vi "Main.vi"() -> ()   [LabVIEW 2021] (continued)
                n259 = Two Button Dialog(message="确定修改？" ("消息")) -> (T button?=w366:bool)  [unwired: 2 in]
                n260 = local read "控件配置文件"() -> (w364:string[][])
                n261 = property on="表格" class="Tbl (严格)"() -> ("Value"=w363:string[][])  [unwired: 2 in, 2 out]
                n262 = call "设控值写入.vi"("表格"=w363, "控件配置文件"=w364, "DataInitDef"=w361, "NewVal"=w365, "布尔"=w366) -> ("输出簇"=w362:cluster{u16, i32, i32, i32})  [unwired: 10 in]
                n263 = property on="要发送的数据" class="Clust (严格)"("Val(Sgnl)"=w362) -> ()  [unwired: 2 in, 2 out]
              }
              event "设控2": Value Change {
                w368 = T9 23 items=["刷新间隔", "波特率", "布尔1设置项", "布尔2设置项", "布尔3设置项", "布尔4设置项", "布尔5设置项", "布尔6设置项", "布尔7设置项", "布尔8设置项", "显控1设置", "显控2设置", "显控3设置", "显控4设置", "显控5设置", "显控6设置", "显控7设置", "显控8设置", "显控9设置", "显控10设置", "显控11设置", "显控12设置", "设控1设置", "设控2设置", "设控3设置", "设控4设置", "设控5设置", "设控6设置", "设控7设置", "设控8设置", "曲线1设置", "曲线2设置", "曲线3设置", "曲线4设置", "曲线5设置", "曲线6设置", "曲线7设置", "曲线8设置", "曲线9设置", "曲线10设置", "曲线11设置", "曲线12设置", "曲线13设置", "曲线14设置", "曲线15设置", "曲线16设置", "曲线17设置", "曲线18设置", "曲线19设置", "曲线20设置", "曲线21设置", "曲线22设置", "曲线23设置", "曲线24设置", "曲线25设置", "曲线26设置", "曲线27设置", "曲线28设置", "曲线29设置", "曲线30设置", "曲线31设置", "曲线32设置", "曲线33设置", "曲线34设置", "曲线35设置", "曲线36设置", "曲线37设置", "曲线38设置", "曲线39设置", "曲线40设置", "曲线41设置", "曲线42设置", "曲线43设置", "曲线44设置", "曲线45设置", "曲线46设置", "曲线47设置", "曲线48设置", "曲线49设置", "曲线50设置", "曲线51设置", "曲线52设置", "曲线53设置", "曲线54设置", "曲线55设置", "曲线56设置", "曲线57设置", "曲线58设置", "曲线59设置", "曲线60设置", "曲线61设置", "曲线62设置", "曲线63设置", "曲线64设置", "ID值", "数据模式"] ("DataInitDef")
                n264 = event-data() -> ("NewVal"=w370:string)  [unwired: 1 in, 5 out]
                n265 = Two Button Dialog(message="确定修改？" ("消息")) -> (T button?=w369:bool)  [unwired: 2 in]
                n266 = local read "控件配置文件"() -> (w371:string[][])
                n267 = property on="表格" class="Tbl (严格)"() -> ("Value"=w372:string[][])  [unwired: 2 in, 2 out]
                n268 = call "设控值写入.vi"("表格"=w372, "控件配置文件"=w371, "DataInitDef"=w368, "NewVal"=w370, "布尔"=w369) -> ("输出簇"=w373:cluster{u16, i32, i32, i32})  [unwired: 10 in]
                n269 = property on="要发送的数据" class="Clust (严格)"("Val(Sgnl)"=w373) -> ()  [unwired: 2 in, 2 out]
              }
              event "设控3": Value Change {
                w375 = T9 24 items=["刷新间隔", "波特率", "布尔1设置项", "布尔2设置项", "布尔3设置项", "布尔4设置项", "布尔5设置项", "布尔6设置项", "布尔7设置项", "布尔8设置项", "显控1设置", "显控2设置", "显控3设置", "显控4设置", "显控5设置", "显控6设置", "显控7设置", "显控8设置", "显控9设置", "显控10设置", "显控11设置", "显控12设置", "设控1设置", "设控2设置", "设控3设置", "设控4设置", "设控5设置", "设控6设置", "设控7设置", "设控8设置", "曲线1设置", "曲线2设置", "曲线3设置", "曲线4设置", "曲线5设置", "曲线6设置", "曲线7设置", "曲线8设置", "曲线9设置", "曲线10设置", "曲线11设置", "曲线12设置", "曲线13设置", "曲线14设置", "曲线15设置", "曲线16设置", "曲线17设置", "曲线18设置", "曲线19设置", "曲线20设置", "曲线21设置", "曲线22设置", "曲线23设置", "曲线24设置", "曲线25设置", "曲线26设置", "曲线27设置", "曲线28设置", "曲线29设置", "曲线30设置", "曲线31设置", "曲线32设置", "曲线33设置", "曲线34设置", "曲线35设置", "曲线36设置", "曲线37设置", "曲线38设置", "曲线39设置", "曲线40设置", "曲线41设置", "曲线42设置", "曲线43设置", "曲线44设置", "曲线45设置", "曲线46设置", "曲线47设置", "曲线48设置", "曲线49设置", "曲线50设置", "曲线51设置", "曲线52设置", "曲线53设置", "曲线54设置", "曲线55设置", "曲线56设置", "曲线57设置", "曲线58设置", "曲线59设置", "曲线60设置", "曲线61设置", "曲线62设置", "曲线63设置", "曲线64设置", "ID值", "数据模式"] ("DataInitDef")
                n270 = event-data() -> ("NewVal"=w378:string)  [unwired: 1 in, 5 out]
                n271 = Two Button Dialog(message="确定修改？" ("消息")) -> (T button?=w377:bool)  [unwired: 2 in]
                n272 = local read "控件配置文件"() -> (w379:string[][])
                n273 = property on="表格" class="Tbl (严格)"() -> ("Value"=w380:string[][])  [unwired: 2 in, 2 out]
                n274 = call "设控值写入.vi"("表格"=w380, "控件配置文件"=w379, "DataInitDef"=w375, "NewVal"=w378, "布尔"=w377) -> ("输出簇"=w376:cluster{u16, i32, i32, i32})  [unwired: 10 in]
                n275 = property on="要发送的数据" class="Clust (严格)"("Val(Sgnl)"=w376) -> ()  [unwired: 2 in, 2 out]
              }
              event "设控4": Value Change {
                w382 = T9 25 items=["刷新间隔", "波特率", "布尔1设置项", "布尔2设置项", "布尔3设置项", "布尔4设置项", "布尔5设置项", "布尔6设置项", "布尔7设置项", "布尔8设置项", "显控1设置", "显控2设置", "显控3设置", "显控4设置", "显控5设置", "显控6设置", "显控7设置", "显控8设置", "显控9设置", "显控10设置", "显控11设置", "显控12设置", "设控1设置", "设控2设置", "设控3设置", "设控4设置", "设控5设置", "设控6设置", "设控7设置", "设控8设置", "曲线1设置", "曲线2设置", "曲线3设置", "曲线4设置", "曲线5设置", "曲线6设置", "曲线7设置", "曲线8设置", "曲线9设置", "曲线10设置", "曲线11设置", "曲线12设置", "曲线13设置", "曲线14设置", "曲线15设置", "曲线16设置", "曲线17设置", "曲线18设置", "曲线19设置", "曲线20设置", "曲线21设置", "曲线22设置", "曲线23设置", "曲线24设置", "曲线25设置", "曲线26设置", "曲线27设置", "曲线28设置", "曲线29设置", "曲线30设置", "曲线31设置", "曲线32设置", "曲线33设置", "曲线34设置", "曲线35设置", "曲线36设置", "曲线37设置", "曲线38设置", "曲线39设置", "曲线40设置", "曲线41设置", "曲线42设置", "曲线43设置", "曲线44设置", "曲线45设置", "曲线46设置", "曲线47设置", "曲线48设置", "曲线49设置", "曲线50设置", "曲线51设置", "曲线52设置", "曲线53设置", "曲线54设置", "曲线55设置", "曲线56设置", "曲线57设置", "曲线58设置", "曲线59设置", "曲线60设置", "曲线61设置", "曲线62设置", "曲线63设置", "曲线64设置", "ID值", "数据模式"] ("DataInitDef")
                n276 = event-data() -> ("NewVal"=w385:string)  [unwired: 1 in, 5 out]
                n277 = Two Button Dialog(message="确定修改？" ("消息")) -> (T button?=w384:bool)  [unwired: 2 in]
                n278 = local read "控件配置文件"() -> (w386:string[][])
                n279 = property on="表格" class="Tbl (严格)"() -> ("Value"=w387:string[][])  [unwired: 2 in, 2 out]
                n280 = call "设控值写入.vi"("表格"=w387, "控件配置文件"=w386, "DataInitDef"=w382, "NewVal"=w385, "布尔"=w384) -> ("输出簇"=w383:cluster{u16, i32, i32, i32})  [unwired: 10 in]
                n281 = property on="要发送的数据" class="Clust (严格)"("Val(Sgnl)"=w383) -> ()  [unwired: 2 in, 2 out]
              }
              event "设控5": Value Change {
                w389 = T9 26 items=["刷新间隔", "波特率", "布尔1设置项", "布尔2设置项", "布尔3设置项", "布尔4设置项", "布尔5设置项", "布尔6设置项", "布尔7设置项", "布尔8设置项", "显控1设置", "显控2设置", "显控3设置", "显控4设置", "显控5设置", "显控6设置", "显控7设置", "显控8设置", "显控9设置", "显控10设置", "显控11设置", "显控12设置", "设控1设置", "设控2设置", "设控3设置", "设控4设置", "设控5设置", "设控6设置", "设控7设置", "设控8设置", "曲线1设置", "曲线2设置", "曲线3设置", "曲线4设置", "曲线5设置", "曲线6设置", "曲线7设置", "曲线8设置", "曲线9设置", "曲线10设置", "曲线11设置", "曲线12设置", "曲线13设置", "曲线14设置", "曲线15设置", "曲线16设置", "曲线17设置", "曲线18设置", "曲线19设置", "曲线20设置", "曲线21设置", "曲线22设置", "曲线23设置", "曲线24设置", "曲线25设置", "曲线26设置", "曲线27设置", "曲线28设置", "曲线29设置", "曲线30设置", "曲线31设置", "曲线32设置", "曲线33设置", "曲线34设置", "曲线35设置", "曲线36设置", "曲线37设置", "曲线38设置", "曲线39设置", "曲线40设置", "曲线41设置", "曲线42设置", "曲线43设置", "曲线44设置", "曲线45设置", "曲线46设置", "曲线47设置", "曲线48设置", "曲线49设置", "曲线50设置", "曲线51设置", "曲线52设置", "曲线53设置", "曲线54设置", "曲线55设置", "曲线56设置", "曲线57设置", "曲线58设置", "曲线59设置", "曲线60设置", "曲线61设置", "曲线62设置", "曲线63设置", "曲线64设置", "ID值", "数据模式"] ("DataInitDef")
                n282 = event-data() -> ("NewVal"=w391:string)  [unwired: 1 in, 5 out]
                n283 = Two Button Dialog(message="确定修改？" ("消息")) -> (T button?=w390:bool)  [unwired: 2 in]
                n284 = local read "控件配置文件"() -> (w392:string[][])
                n285 = property on="表格" class="Tbl (严格)"() -> ("Value"=w393:string[][])  [unwired: 2 in, 2 out]
                n286 = call "设控值写入.vi"("表格"=w393, "控件配置文件"=w392, "DataInitDef"=w389, "NewVal"=w391, "布尔"=w390) -> ("输出簇"=w394:cluster{u16, i32, i32, i32})  [unwired: 10 in]
                n287 = property on="要发送的数据" class="Clust (严格)"("Val(Sgnl)"=w394) -> ()  [unwired: 2 in, 2 out]
              }
              event "设控6": Value Change {
                w396 = T9 27 items=["刷新间隔", "波特率", "布尔1设置项", "布尔2设置项", "布尔3设置项", "布尔4设置项", "布尔5设置项", "布尔6设置项", "布尔7设置项", "布尔8设置项", "显控1设置", "显控2设置", "显控3设置", "显控4设置", "显控5设置", "显控6设置", "显控7设置", "显控8设置", "显控9设置", "显控10设置", "显控11设置", "显控12设置", "设控1设置", "设控2设置", "设控3设置", "设控4设置", "设控5设置", "设控6设置", "设控7设置", "设控8设置", "曲线1设置", "曲线2设置", "曲线3设置", "曲线4设置", "曲线5设置", "曲线6设置", "曲线7设置", "曲线8设置", "曲线9设置", "曲线10设置", "曲线11设置", "曲线12设置", "曲线13设置", "曲线14设置", "曲线15设置", "曲线16设置", "曲线17设置", "曲线18设置", "曲线19设置", "曲线20设置", "曲线21设置", "曲线22设置", "曲线23设置", "曲线24设置", "曲线25设置", "曲线26设置", "曲线27设置", "曲线28设置", "曲线29设置", "曲线30设置", "曲线31设置", "曲线32设置", "曲线33设置", "曲线34设置", "曲线35设置", "曲线36设置", "曲线37设置", "曲线38设置", "曲线39设置", "曲线40设置", "曲线41设置", "曲线42设置", "曲线43设置", "曲线44设置", "曲线45设置", "曲线46设置", "曲线47设置", "曲线48设置", "曲线49设置", "曲线50设置", "曲线51设置", "曲线52设置", "曲线53设置", "曲线54设置", "曲线55设置", "曲线56设置", "曲线57设置", "曲线58设置", "曲线59设置", "曲线60设置", "曲线61设置", "曲线62设置", "曲线63设置", "曲线64设置", "ID值", "数据模式"] ("DataInitDef")
                n288 = event-data() -> ("NewVal"=w398:string)  [unwired: 1 in, 5 out]
                n289 = Two Button Dialog(message="确定修改？" ("消息")) -> (T button?=w397:bool)  [unwired: 2 in]
                n290 = local read "控件配置文件"() -> (w399:string[][])
                n291 = property on="表格" class="Tbl (严格)"() -> ("Value"=w400:string[][])  [unwired: 2 in, 2 out]
                n292 = call "设控值写入.vi"("表格"=w400, "控件配置文件"=w399, "DataInitDef"=w396, "NewVal"=w398, "布尔"=w397) -> ("输出簇"=w401:cluster{u16, i32, i32, i32})  [unwired: 10 in]
                n293 = property on="要发送的数据" class="Clust (严格)"("Val(Sgnl)"=w401) -> ()  [unwired: 2 in, 2 out]
              }
              event "设控7": Value Change {
                w403 = T9 28 items=["刷新间隔", "波特率", "布尔1设置项", "布尔2设置项", "布尔3设置项", "布尔4设置项", "布尔5设置项", "布尔6设置项", "布尔7设置项", "布尔8设置项", "显控1设置", "显控2设置", "显控3设置", "显控4设置", "显控5设置", "显控6设置", "显控7设置", "显控8设置", "显控9设置", "显控10设置", "显控11设置", "显控12设置", "设控1设置", "设控2设置", "设控3设置", "设控4设置", "设控5设置", "设控6设置", "设控7设置", "设控8设置", "曲线1设置", "曲线2设置", "曲线3设置", "曲线4设置", "曲线5设置", "曲线6设置", "曲线7设置", "曲线8设置", "曲线9设置", "曲线10设置", "曲线11设置", "曲线12设置", "曲线13设置", "曲线14设置", "曲线15设置", "曲线16设置", "曲线17设置", "曲线18设置", "曲线19设置", "曲线20设置", "曲线21设置", "曲线22设置", "曲线23设置", "曲线24设置", "曲线25设置", "曲线26设置", "曲线27设置", "曲线28设置", "曲线29设置", "曲线30设置", "曲线31设置", "曲线32设置", "曲线33设置", "曲线34设置", "曲线35设置", "曲线36设置", "曲线37设置", "曲线38设置", "曲线39设置", "曲线40设置", "曲线41设置", "曲线42设置", "曲线43设置", "曲线44设置", "曲线45设置", "曲线46设置", "曲线47设置", "曲线48设置", "曲线49设置", "曲线50设置", "曲线51设置", "曲线52设置", "曲线53设置", "曲线54设置", "曲线55设置", "曲线56设置", "曲线57设置", "曲线58设置", "曲线59设置", "曲线60设置", "曲线61设置", "曲线62设置", "曲线63设置", "曲线64设置", "ID值", "数据模式"] ("DataInitDef")
                n294 = event-data() -> ("NewVal"=w405:string)  [unwired: 1 in, 5 out]
                n295 = Two Button Dialog(message="确定修改？" ("消息")) -> (T button?=w404:bool)  [unwired: 2 in]
                n296 = local read "控件配置文件"() -> (w406:string[][])
                n297 = property on="表格" class="Tbl (严格)"() -> ("Value"=w407:string[][])  [unwired: 2 in, 2 out]
                n298 = call "设控值写入.vi"("表格"=w407, "控件配置文件"=w406, "DataInitDef"=w403, "NewVal"=w405, "布尔"=w404) -> ("输出簇"=w408:cluster{u16, i32, i32, i32})  [unwired: 10 in]
                n299 = property on="要发送的数据" class="Clust (严格)"("Val(Sgnl)"=w408) -> ()  [unwired: 2 in, 2 out]
              }
              event "设控8": Value Change {
                w410 = T9 29 items=["刷新间隔", "波特率", "布尔1设置项", "布尔2设置项", "布尔3设置项", "布尔4设置项", "布尔5设置项", "布尔6设置项", "布尔7设置项", "布尔8设置项", "显控1设置", "显控2设置", "显控3设置", "显控4设置", "显控5设置", "显控6设置", "显控7设置", "显控8设置", "显控9设置", "显控10设置", "显控11设置", "显控12设置", "设控1设置", "设控2设置", "设控3设置", "设控4设置", "设控5设置", "设控6设置", "设控7设置", "设控8设置", "曲线1设置", "曲线2设置", "曲线3设置", "曲线4设置", "曲线5设置", "曲线6设置", "曲线7设置", "曲线8设置", "曲线9设置", "曲线10设置", "曲线11设置", "曲线12设置", "曲线13设置", "曲线14设置", "曲线15设置", "曲线16设置", "曲线17设置", "曲线18设置", "曲线19设置", "曲线20设置", "曲线21设置", "曲线22设置", "曲线23设置", "曲线24设置", "曲线25设置", "曲线26设置", "曲线27设置", "曲线28设置", "曲线29设置", "曲线30设置", "曲线31设置", "曲线32设置", "曲线33设置", "曲线34设置", "曲线35设置", "曲线36设置", "曲线37设置", "曲线38设置", "曲线39设置", "曲线40设置", "曲线41设置", "曲线42设置", "曲线43设置", "曲线44设置", "曲线45设置", "曲线46设置", "曲线47设置", "曲线48设置", "曲线49设置", "曲线50设置", "曲线51设置", "曲线52设置", "曲线53设置", "曲线54设置", "曲线55设置", "曲线56设置", "曲线57设置", "曲线58设置", "曲线59设置", "曲线60设置", "曲线61设置", "曲线62设置", "曲线63设置", "曲线64设置", "ID值", "数据模式"] ("DataInitDef")
                n300 = event-data() -> ("NewVal"=w412:string)  [unwired: 1 in, 5 out]
                n301 = Two Button Dialog(message="确定修改？" ("消息")) -> (T button?=w411:bool)  [unwired: 2 in]
                n302 = local read "控件配置文件"() -> (w413:string[][])
                n303 = property on="表格" class="Tbl (严格)"() -> ("Value"=w414:string[][])  [unwired: 2 in, 2 out]
                n304 = call "设控值写入.vi"("表格"=w414, "控件配置文件"=w413, "DataInitDef"=w410, "NewVal"=w412, "布尔"=w411) -> ("输出簇"=w415:cluster{u16, i32, i32, i32})  [unwired: 10 in]
                n305 = property on="要发送的数据" class="Clust (严格)"("Val(Sgnl)"=w415) -> ()  [unwired: 2 in, 2 out]
              }
              event "布尔 2": Value Change {
                w417 = T9 3 items=["刷新间隔", "波特率", "布尔1设置项", "布尔2设置项", "布尔3设置项", "布尔4设置项", "布尔5设置项", "布尔6设置项", "布尔7设置项", "布尔8设置项", "显控1设置", "显控2设置", "显控3设置", "显控4设置", "显控5设置", "显控6设置", "显控7设置", "显控8设置", "显控9设置", "显控10设置", "显控11设置", "显控12设置", "设控1设置", "设控2设置", "设控3设置", "设控4设置", "设控5设置", "设控6设置", "设控7设置", "设控8设置", "曲线1设置", "曲线2设置", "曲线3设置", "曲线4设置", "曲线5设置", "曲线6设置", "曲线7设置", "曲线8设置", "曲线9设置", "曲线10设置", "曲线11设置", "曲线12设置", "曲线13设置", "曲线14设置", "曲线15设置", "曲线16设置", "曲线17设置", "曲线18设置", "曲线19设置", "曲线20设置", "曲线21设置", "曲线22设置", "曲线23设置", "曲线24设置", "曲线25设置", "曲线26设置", "曲线27设置", "曲线28设置", "曲线29设置", "曲线30设置", "曲线31设置", "曲线32设置", "曲线33设置", "曲线34设置", "曲线35设置", "曲线36设置", "曲线37设置", "曲线38设置", "曲线39设置", "曲线40设置", "曲线41设置", "曲线42设置", "曲线43设置", "曲线44设置", "曲线45设置", "曲线46设置", "曲线47设置", "曲线48设置", "曲线49设置", "曲线50设置", "曲线51设置", "曲线52设置", "曲线53设置", "曲线54设置", "曲线55设置", "曲线56设置", "曲线57设置", "曲线58设置", "曲线59设置", "曲线60设置", "曲线61设置", "曲线62设置", "曲线63设置", "曲线64设置", "ID值", "数据模式"] ("DataInitDef")
                n306 = event-data() -> ("NewVal"=w418:bool)  [unwired: 1 in]
                n307 = local read "控件配置文件"() -> (w424:string[][])
                n308 = Index Array(array=w424, index (row)=w417, index (col)=1 ("禁用的索引 (列)")) -> (element=w423:string)
                n309 = Not Equal?(x=w423, y="") -> (x != y?=w420:bool)
                n310 = Not Equal?(x=w423, y="X") -> (x != y?=w419:bool)
                n311 = And(x=w420, y=w419) -> (x .and. y?=w421:bool)
                n312 = case shown="真" w421 {
                  tunnel: w418 -> [_ w428]
                  tunnel: w423 -> [_ w429]
                  frame False {
                  }
                  frame True {
                    n313 = local write "延时更新布尔状态"(i16 0 ("延时更新布尔状态")) -> ()
                    n314 = property on="表格" class="Tbl (严格)"() -> ("Value"=w430:string[][])  [unwired: 2 in, 2 out]
                    n315 = call "布尔数据处理.vi"("布尔输入"=w428, "行数"=w429, "表格"=w430) -> ("要发送的数据"=w427:cluster{"地址":u16, "数据":i32, "行数":i32, "ID":i32})  [unwired: 8 in]
                    n316 = property on="要发送的数据" class="Clust (严格)"("Val(Sgnl)"=w427) -> ()  [unwired: 2 in, 2 out]
                  }
                }
              }
              event "布尔 3": Value Change {
                w432 = T9 4 items=["刷新间隔", "波特率", "布尔1设置项", "布尔2设置项", "布尔3设置项", "布尔4设置项", "布尔5设置项", "布尔6设置项", "布尔7设置项", "布尔8设置项", "显控1设置", "显控2设置", "显控3设置", "显控4设置", "显控5设置", "显控6设置", "显控7设置", "显控8设置", "显控9设置", "显控10设置", "显控11设置", "显控12设置", "设控1设置", "设控2设置", "设控3设置", "设控4设置", "设控5设置", "设控6设置", "设控7设置", "设控8设置", "曲线1设置", "曲线2设置", "曲线3设置", "曲线4设置", "曲线5设置", "曲线6设置", "曲线7设置", "曲线8设置", "曲线9设置", "曲线10设置", "曲线11设置", "曲线12设置", "曲线13设置", "曲线14设置", "曲线15设置", "曲线16设置", "曲线17设置", "曲线18设置", "曲线19设置", "曲线20设置", "曲线21设置", "曲线22设置", "曲线23设置", "曲线24设置", "曲线25设置", "曲线26设置", "曲线27设置", "曲线28设置", "曲线29设置", "曲线30设置", "曲线31设置", "曲线32设置", "曲线33设置", "曲线34设置", "曲线35设置", "曲线36设置", "曲线37设置", "曲线38设置", "曲线39设置", "曲线40设置", "曲线41设置", "曲线42设置", "曲线43设置", "曲线44设置", "曲线45设置", "曲线46设置", "曲线47设置", "曲线48设置", "曲线49设置", "曲线50设置", "曲线51设置", "曲线52设置", "曲线53设置", "曲线54设置", "曲线55设置", "曲线56设置", "曲线57设置", "曲线58设置", "曲线59设置", "曲线60设置", "曲线61设置", "曲线62设置", "曲线63设置", "曲线64设置", "ID值", "数据模式"] ("DataInitDef")
                n317 = event-data() -> ("NewVal"=w433:bool)  [unwired: 1 in]
                n318 = local read "控件配置文件"() -> (w439:string[][])
                n319 = Index Array(array=w439, index (row)=w432, index (col)=1 ("禁用的索引 (列)")) -> (element=w438:string)
                n320 = Not Equal?(x=w438, y="") -> (x != y?=w435:bool)
                n321 = Not Equal?(x=w438, y="X") -> (x != y?=w434:bool)
                n322 = And(x=w435, y=w434) -> (x .and. y?=w436:bool)
                n323 = case shown="真" w436 {
                  tunnel: w438 -> [_ w444]
                  tunnel: w433 -> [_ w443]
                  frame False {
                  }
                  frame True {
                    n324 = local write "延时更新布尔状态"(i16 0 ("延时更新布尔状态")) -> ()
                    n325 = property on="表格" class="Tbl (严格)"() -> ("Value"=w445:string[][])  [unwired: 2 in, 2 out]
                    n326 = call "布尔数据处理.vi"("布尔输入"=w443, "行数"=w444, "表格"=w445) -> ("要发送的数据"=w442:cluster{"地址":u16, "数据":i32, "行数":i32, "ID":i32})  [unwired: 8 in]
                    n327 = property on="要发送的数据" class="Clust (严格)"("Val(Sgnl)"=w442) -> ()  [unwired: 2 in, 2 out]
                  }
                }
              }
              event "布尔 4": Value Change {
                w447 = T9 5 items=["刷新间隔", "波特率", "布尔1设置项", "布尔2设置项", "布尔3设置项", "布尔4设置项", "布尔5设置项", "布尔6设置项", "布尔7设置项", "布尔8设置项", "显控1设置", "显控2设置", "显控3设置", "显控4设置", "显控5设置", "显控6设置", "显控7设置", "显控8设置", "显控9设置", "显控10设置", "显控11设置", "显控12设置", "设控1设置", "设控2设置", "设控3设置", "设控4设置", "设控5设置", "设控6设置", "设控7设置", "设控8设置", "曲线1设置", "曲线2设置", "曲线3设置", "曲线4设置", "曲线5设置", "曲线6设置", "曲线7设置", "曲线8设置", "曲线9设置", "曲线10设置", "曲线11设置", "曲线12设置", "曲线13设置", "曲线14设置", "曲线15设置", "曲线16设置", "曲线17设置", "曲线18设置", "曲线19设置", "曲线20设置", "曲线21设置", "曲线22设置", "曲线23设置", "曲线24设置", "曲线25设置", "曲线26设置", "曲线27设置", "曲线28设置", "曲线29设置", "曲线30设置", "曲线31设置", "曲线32设置", "曲线33设置", "曲线34设置", "曲线35设置", "曲线36设置", "曲线37设置", "曲线38设置", "曲线39设置", "曲线40设置", "曲线41设置", "曲线42设置", "曲线43设置", "曲线44设置", "曲线45设置", "曲线46设置", "曲线47设置", "曲线48设置", "曲线49设置", "曲线50设置", "曲线51设置", "曲线52设置", "曲线53设置", "曲线54设置", "曲线55设置", "曲线56设置", "曲线57设置", "曲线58设置", "曲线59设置", "曲线60设置", "曲线61设置", "曲线62设置", "曲线63设置", "曲线64设置", "ID值", "数据模式"] ("DataInitDef")
                n328 = event-data() -> ("NewVal"=w448:bool)  [unwired: 1 in]
                n329 = local read "控件配置文件"() -> (w456:string[][])
                n330 = Index Array(array=w456, index (row)=w447, index (col)=1 ("禁用的索引 (列)")) -> (element=w455:string)
                n331 = Not Equal?(x=w455, y="") -> (x != y?=w453:bool)
                n332 = Not Equal?(x=w455, y="X") -> (x != y?=w452:bool)
                n333 = And(x=w453, y=w452) -> (x .and. y?=w454:bool)
                n334 = case shown="真" w454 {
                  tunnel: w448 -> [_ w458]
                  tunnel: w455 -> [_ w459]
                  frame False {
                  }
                  frame True {
                    n335 = local write "延时更新布尔状态"(i16 0 ("延时更新布尔状态")) -> ()
                    n336 = property on="表格" class="Tbl (严格)"() -> ("Value"=w460:string[][])  [unwired: 2 in, 2 out]
                    n337 = call "布尔数据处理.vi"("布尔输入"=w458, "行数"=w459, "表格"=w460) -> ("要发送的数据"=w457:cluster{"地址":u16, "数据":i32, "行数":i32, "ID":i32})  [unwired: 8 in]
                    n338 = property on="要发送的数据" class="Clust (严格)"("Val(Sgnl)"=w457) -> ()  [unwired: 2 in, 2 out]
                  }
                }
              }
              event "布尔 5": Value Change {
                w462 = T9 6 items=["刷新间隔", "波特率", "布尔1设置项", "布尔2设置项", "布尔3设置项", "布尔4设置项", "布尔5设置项", "布尔6设置项", "布尔7设置项", "布尔8设置项", "显控1设置", "显控2设置", "显控3设置", "显控4设置", "显控5设置", "显控6设置", "显控7设置", "显控8设置", "显控9设置", "显控10设置", "显控11设置", "显控12设置", "设控1设置", "设控2设置", "设控3设置", "设控4设置", "设控5设置", "设控6设置", "设控7设置", "设控8设置", "曲线1设置", "曲线2设置", "曲线3设置", "曲线4设置", "曲线5设置", "曲线6设置", "曲线7设置", "曲线8设置", "曲线9设置", "曲线10设置", "曲线11设置", "曲线12设置", "曲线13设置", "曲线14设置", "曲线15设置", "曲线16设置", "曲线17设置", "曲线18设置", "曲线19设置", "曲线20设置", "曲线21设置", "曲线22设置", "曲线23设置", "曲线24设置", "曲线25设置", "曲线26设置", "曲线27设置", "曲线28设置", "曲线29设置", "曲线30设置", "曲线31设置", "曲线32设置", "曲线33设置", "曲线34设置", "曲线35设置", "曲线36设置", "曲线37设置", "曲线38设置", "曲线39设置", "曲线40设置", "曲线41设置", "曲线42设置", "曲线43设置", "曲线44设置", "曲线45设置", "曲线46设置", "曲线47设置", "曲线48设置", "曲线49设置", "曲线50设置", "曲线51设置", "曲线52设置", "曲线53设置", "曲线54设置", "曲线55设置", "曲线56设置", "曲线57设置", "曲线58设置", "曲线59设置", "曲线60设置", "曲线61设置", "曲线62设置", "曲线63设置", "曲线64设置", "ID值", "数据模式"] ("DataInitDef")
                n339 = event-data() -> ("NewVal"=w463:bool)  [unwired: 1 in]
                n340 = local read "控件配置文件"() -> (w471:string[][])
                n341 = Index Array(array=w471, index (row)=w462, index (col)=1 ("禁用的索引 (列)")) -> (element=w470:string)
                n342 = Not Equal?(x=w470, y="") -> (x != y?=w468:bool)
                n343 = Not Equal?(x=w470, y="X") -> (x != y?=w467:bool)
                n344 = And(x=w468, y=w467) -> (x .and. y?=w469:bool)
                n345 = case shown="真" w469 {
                  tunnel: w463 -> [_ w473]
                  tunnel: w470 -> [_ w474]
                  frame False {
                  }
                  frame True {
                    n346 = local write "延时更新布尔状态"(i16 0 ("延时更新布尔状态")) -> ()
                    n347 = property on="表格" class="Tbl (严格)"() -> ("Value"=w475:string[][])  [unwired: 2 in, 2 out]
                    n348 = call "布尔数据处理.vi"("布尔输入"=w473, "行数"=w474, "表格"=w475) -> ("要发送的数据"=w472:cluster{"地址":u16, "数据":i32, "行数":i32, "ID":i32})  [unwired: 8 in]
                    n349 = property on="要发送的数据" class="Clust (严格)"("Val(Sgnl)"=w472) -> ()  [unwired: 2 in, 2 out]
                  }
                }
              }
              event "布尔 6": Value Change {
                w477 = T9 7 items=["刷新间隔", "波特率", "布尔1设置项", "布尔2设置项", "布尔3设置项", "布尔4设置项", "布尔5设置项", "布尔6设置项", "布尔7设置项", "布尔8设置项", "显控1设置", "显控2设置", "显控3设置", "显控4设置", "显控5设置", "显控6设置", "显控7设置", "显控8设置", "显控9设置", "显控10设置", "显控11设置", "显控12设置", "设控1设置", "设控2设置", "设控3设置", "设控4设置", "设控5设置", "设控6设置", "设控7设置", "设控8设置", "曲线1设置", "曲线2设置", "曲线3设置", "曲线4设置", "曲线5设置", "曲线6设置", "曲线7设置", "曲线8设置", "曲线9设置", "曲线10设置", "曲线11设置", "曲线12设置", "曲线13设置", "曲线14设置", "曲线15设置", "曲线16设置", "曲线17设置", "曲线18设置", "曲线19设置", "曲线20设置", "曲线21设置", "曲线22设置", "曲线23设置", "曲线24设置", "曲线25设置", "曲线26设置", "曲线27设置", "曲线28设置", "曲线29设置", "曲线30设置", "曲线31设置", "曲线32设置", "曲线33设置", "曲线34设置", "曲线35设置", "曲线36设置", "曲线37设置", "曲线38设置", "曲线39设置", "曲线40设置", "曲线41设置", "曲线42设置", "曲线43设置", "曲线44设置", "曲线45设置", "曲线46设置", "曲线47设置", "曲线48设置", "曲线49设置", "曲线50设置", "曲线51设置", "曲线52设置", "曲线53设置", "曲线54设置", "曲线55设置", "曲线56设置", "曲线57设置", "曲线58设置", "曲线59设置", "曲线60设置", "曲线61设置", "曲线62设置", "曲线63设置", "曲线64设置", "ID值", "数据模式"] ("DataInitDef")
                n350 = event-data() -> ("NewVal"=w478:bool)  [unwired: 1 in]
                n351 = local read "控件配置文件"() -> (w486:string[][])
                n352 = Index Array(array=w486, index (row)=w477, index (col)=1 ("禁用的索引 (列)")) -> (element=w485:string)
                n353 = Not Equal?(x=w485, y="") -> (x != y?=w483:bool)
                n354 = Not Equal?(x=w485, y="X") -> (x != y?=w482:bool)
                n355 = And(x=w483, y=w482) -> (x .and. y?=w484:bool)
                n356 = case shown="真" w484 {
                  tunnel: w478 -> [_ w488]
                  tunnel: w485 -> [_ w489]
                  frame False {
                  }
                  frame True {
                    n357 = local write "延时更新布尔状态"(i16 0 ("延时更新布尔状态")) -> ()
                    n358 = property on="表格" class="Tbl (严格)"() -> ("Value"=w490:string[][])  [unwired: 2 in, 2 out]
                    n359 = call "布尔数据处理.vi"("布尔输入"=w488, "行数"=w489, "表格"=w490) -> ("要发送的数据"=w487:cluster{"地址":u16, "数据":i32, "行数":i32, "ID":i32})  [unwired: 8 in]
                    n360 = property on="要发送的数据" class="Clust (严格)"("Val(Sgnl)"=w487) -> ()  [unwired: 2 in, 2 out]
                  }
                }
              }
              event "布尔 7": Value Change {
                w492 = T9 8 items=["刷新间隔", "波特率", "布尔1设置项", "布尔2设置项", "布尔3设置项", "布尔4设置项", "布尔5设置项", "布尔6设置项", "布尔7设置项", "布尔8设置项", "显控1设置", "显控2设置", "显控3设置", "显控4设置", "显控5设置", "显控6设置", "显控7设置", "显控8设置", "显控9设置", "显控10设置", "显控11设置", "显控12设置", "设控1设置", "设控2设置", "设控3设置", "设控4设置", "设控5设置", "设控6设置", "设控7设置", "设控8设置", "曲线1设置", "曲线2设置", "曲线3设置", "曲线4设置", "曲线5设置", "曲线6设置", "曲线7设置", "曲线8设置", "曲线9设置", "曲线10设置", "曲线11设置", "曲线12设置", "曲线13设置", "曲线14设置", "曲线15设置", "曲线16设置", "曲线17设置", "曲线18设置", "曲线19设置", "曲线20设置", "曲线21设置", "曲线22设置", "曲线23设置", "曲线24设置", "曲线25设置", "曲线26设置", "曲线27设置", "曲线28设置", "曲线29设置", "曲线30设置", "曲线31设置", "曲线32设置", "曲线33设置", "曲线34设置", "曲线35设置", "曲线36设置", "曲线37设置", "曲线38设置", "曲线39设置", "曲线40设置", "曲线41设置", "曲线42设置", "曲线43设置", "曲线44设置", "曲线45设置", "曲线46设置", "曲线47设置", "曲线48设置", "曲线49设置", "曲线50设置", "曲线51设置", "曲线52设置", "曲线53设置", "曲线54设置", "曲线55设置", "曲线56设置", "曲线57设置", "曲线58设置", "曲线59设置", "曲线60设置", "曲线61设置", "曲线62设置", "曲线63设置", "曲线64设置", "ID值", "数据模式"] ("DataInitDef")
                n361 = event-data() -> ("NewVal"=w493:bool)  [unwired: 1 in]
                n362 = local read "控件配置文件"() -> (w501:string[][])
                n363 = Index Array(array=w501, index (row)=w492, index (col)=1 ("禁用的索引 (列)")) -> (element=w500:string)
                n364 = Not Equal?(x=w500, y="") -> (x != y?=w498:bool)
                n365 = Not Equal?(x=w500, y="X") -> (x != y?=w497:bool)
                n366 = And(x=w498, y=w497) -> (x .and. y?=w499:bool)
                n367 = case shown="真" w499 {
                  tunnel: w493 -> [_ w503]
                  tunnel: w500 -> [_ w504]
                  frame False {
                  }
                  frame True {
                    n368 = local write "延时更新布尔状态"(i16 0 ("延时更新布尔状态")) -> ()
                    n369 = property on="表格" class="Tbl (严格)"() -> ("Value"=w505:string[][])  [unwired: 2 in, 2 out]
                    n370 = call "布尔数据处理.vi"("布尔输入"=w503, "行数"=w504, "表格"=w505) -> ("要发送的数据"=w502:cluster{"地址":u16, "数据":i32, "行数":i32, "ID":i32})  [unwired: 8 in]
                    n371 = property on="要发送的数据" class="Clust (严格)"("Val(Sgnl)"=w502) -> ()  [unwired: 2 in, 2 out]
                  }
                }
              }
              event "布尔 8": Value Change {
                w507 = T9 9 items=["刷新间隔", "波特率", "布尔1设置项", "布尔2设置项", "布尔3设置项", "布尔4设置项", "布尔5设置项", "布尔6设置项", "布尔7设置项", "布尔8设置项", "显控1设置", "显控2设置", "显控3设置", "显控4设置", "显控5设置", "显控6设置", "显控7设置", "显控8设置", "显控9设置", "显控10设置", "显控11设置", "显控12设置", "设控1设置", "设控2设置", "设控3设置", "设控4设置", "设控5设置", "设控6设置", "设控7设置", "设控8设置", "曲线1设置", "曲线2设置", "曲线3设置", "曲线4设置", "曲线5设置", "曲线6设置", "曲线7设置", "曲线8设置", "曲线9设置", "曲线10设置", "曲线11设置", "曲线12设置", "曲线13设置", "曲线14设置", "曲线15设置", "曲线16设置", "曲线17设置", "曲线18设置", "曲线19设置", "曲线20设置", "曲线21设置", "曲线22设置", "曲线23设置", "曲线24设置", "曲线25设置", "曲线26设置", "曲线27设置", "曲线28设置", "曲线29设置", "曲线30设置", "曲线31设置", "曲线32设置", "曲线33设置", "曲线34设置", "曲线35设置", "曲线36设置", "曲线37设置", "曲线38设置", "曲线39设置", "曲线40设置", "曲线41设置", "曲线42设置", "曲线43设置", "曲线44设置", "曲线45设置", "曲线46设置", "曲线47设置", "曲线48设置", "曲线49设置", "曲线50设置", "曲线51设置", "曲线52设置", "曲线53设置", "曲线54设置", "曲线55设置", "曲线56设置", "曲线57设置", "曲线58设置", "曲线59设置", "曲线60设置", "曲线61设置", "曲线62设置", "曲线63设置", "曲线64设置", "ID值", "数据模式"] ("DataInitDef")
                n372 = event-data() -> ("NewVal"=w508:bool)  [unwired: 1 in]
                n373 = local read "控件配置文件"() -> (w516:string[][])
                n374 = Index Array(array=w516, index (row)=w507, index (col)=1 ("禁用的索引 (列)")) -> (element=w515:string)
                n375 = Not Equal?(x=w515, y="") -> (x != y?=w513:bool)
                n376 = Not Equal?(x=w515, y="X") -> (x != y?=w512:bool)
                n377 = And(x=w513, y=w512) -> (x .and. y?=w514:bool)
                n378 = case shown="真" w514 {
                  tunnel: w508 -> [_ w518]
                  tunnel: w515 -> [_ w519]
                  frame False {
                  }
                  frame True {
                    n379 = local write "延时更新布尔状态"(i16 0 ("延时更新布尔状态")) -> ()
                    n380 = property on="表格" class="Tbl (严格)"() -> ("Value"=w520:string[][])  [unwired: 2 in, 2 out]
                    n381 = call "布尔数据处理.vi"("布尔输入"=w518, "行数"=w519, "表格"=w520) -> ("要发送的数据"=w517:cluster{"地址":u16, "数据":i32, "行数":i32, "ID":i32})  [unwired: 8 in]
                    n382 = property on="要发送的数据" class="Clust (严格)"("Val(Sgnl)"=w517) -> ()  [unwired: 2 in, 2 out]
                  }
                }
              }
            }
          }
          frame #1 {
            # "处理表格右键关联的代码"
            n383 = event "事件结构" shown="[1] \"表格\": 快捷菜单选择（用户）" {
              selector: _ -> [_ _]
              dyn-events: _ -> [_ _]
              timeout: 0 -> [_ _]
              event Timeout {
                n384 = event-data() -> ()  [unwired: 1 in, 3 out]
              }
              event "表格": Shortcut Menu Selection (User) {
                # "处理关联到布尔控件的代码"
                n385 = event-data() -> ("ItemTag"=w523:string)  [unwired: 1 in, 7 out]
                n386 = case shown="\"关联到设控1\"" w523 {
                  frame "假", Default {
                  }
                  frame "关联到布控1" {
                    w524 = T9 2 items=["刷新间隔", "波特率", "布尔1设置项", "布尔2设置项", "布尔3设置项", "布尔4设置项", "布尔5设置项", "布尔6设置项", "布尔7设置项", "布尔8设置项", "显控1设置", "显控2设置", "显控3设置", "显控4设置", "显控5设置", "显控6设置", "显控7设置", "显控8设置", "显控9设置", "显控10设置", "显控11设置", "显控12设置", "设控1设置", "设控2设置", "设控3设置", "设控4设置", "设控5设置", "设控6设置", "设控7设置", "设控8设置", "曲线1设置", "曲线2设置", "曲线3设置", "曲线4设置", "曲线5设置", "曲线6设置", "曲线7设置", "曲线8设置", "曲线9设置", "曲线10设置", "曲线11设置", "曲线12设置", "曲线13设置", "曲线14设置", "曲线15设置", "曲线16设置", "曲线17设置", "曲线18设置", "曲线19设置", "曲线20设置", "曲线21设置", "曲线22设置", "曲线23设置", "曲线24设置", "曲线25设置", "曲线26设置", "曲线27设置", "曲线28设置", "曲线29设置", "曲线30设置", "曲线31设置", "曲线32设置", "曲线33设置", "曲线34设置", "曲线35设置", "曲线36设置", "曲线37设置", "曲线38设置", "曲线39设置", "曲线40设置", "曲线41设置", "曲线42设置", "曲线43设置", "曲线44设置", "曲线45设置", "曲线46设置", "曲线47设置", "曲线48设置", "曲线49设置", "曲线50设置", "曲线51设置", "曲线52设置", "曲线53设置", "曲线54设置", "曲线55设置", "曲线56设置", "曲线57设置", "曲线58设置", "曲线59设置", "曲线60设置", "曲线61设置", "曲线62设置", "曲线63设置", "曲线64设置", "ID值", "数据模式"] ("DataInitDef")
                    n387 = property on="表格" class="Tbl (严格)"() -> ("Selection Start"=w533:T1)  [unwired: 2 in, 2 out]
                    n388 = Unbundle By Name(w533) -> ("Row"=w529:i32)
                    n389 = property on="表格" class="Tbl (严格)"() -> ("Value"=w534:string[][])  [unwired: 2 in, 2 out]
                    n390 = Number To Decimal String(number=w529) -> (decimal integer string=w528:string)  [unwired: 1 in]
                    n391 = Index Array(array=w534, index (row)=w529, index (col)=0 ("禁用的索引 (列)")) -> (element=w526:string)
                    n392 = String Subset(string=w526, length (rest)=10 ("长度（剩余）")) -> (substring=w525:string)  [unwired: 1 in]
                    n393 = invoke on="控件配置文件" class="Tbl (严格)" method="Set Cell Value"("X Index"=1 ("X索引"), "Y Index"=w524, "Value"=w528) -> ()  [unwired: 3 in, 6 out]
                    n394 = property on="布控1设置" class="Str"("Val(Sgnl)"=w525) -> ()  [unwired: 2 in, 2 out]
                    n395 = property on="布尔 1" class="Bool (严格)"("Caption.Text"=w525) -> ()  [unwired: 2 in, 2 out]
                    n396 = invoke on="控件配置文件" class="Tbl (严格)" method="Set Cell Value"("X Index"=0 ("X索引"), "Y Index"=w524, "Value"=w525) -> ()  [unwired: 3 in, 6 out]
                  }
                  frame "关联到布控2" {
                    w535 = T9 3 items=["刷新间隔", "波特率", "布尔1设置项", "布尔2设置项", "布尔3设置项", "布尔4设置项", "布尔5设置项", "布尔6设置项", "布尔7设置项", "布尔8设置项", "显控1设置", "显控2设置", "显控3设置", "显控4设置", "显控5设置", "显控6设置", "显控7设置", "显控8设置", "显控9设置", "显控10设置", "显控11设置", "显控12设置", "设控1设置", "设控2设置", "设控3设置", "设控4设置", "设控5设置", "设控6设置", "设控7设置", "设控8设置", "曲线1设置", "曲线2设置", "曲线3设置", "曲线4设置", "曲线5设置", "曲线6设置", "曲线7设置", "曲线8设置", "曲线9设置", "曲线10设置", "曲线11设置", "曲线12设置", "曲线13设置", "曲线14设置", "曲线15设置", "曲线16设置", "曲线17设置", "曲线18设置", "曲线19设置", "曲线20设置", "曲线21设置", "曲线22设置", "曲线23设置", "曲线24设置", "曲线25设置", "曲线26设置", "曲线27设置", "曲线28设置", "曲线29设置", "曲线30设置", "曲线31设置", "曲线32设置", "曲线33设置", "曲线34设置", "曲线35设置", "曲线36设置", "曲线37设置", "曲线38设置", "曲线39设置", "曲线40设置", "曲线41设置", "曲线42设置", "曲线43设置", "曲线44设置", "曲线45设置", "曲线46设置", "曲线47设置", "曲线48设置", "曲线49设置", "曲线50设置", "曲线51设置", "曲线52设置", "曲线53设置", "曲线54设置", "曲线55设置", "曲线56设置", "曲线57设置", "曲线58设置", "曲线59设置", "曲线60设置", "曲线61设置", "曲线62设置", "曲线63设置", "曲线64设置", "ID值", "数据模式"] ("DataInitDef")
                    n397 = property on="表格" class="Tbl (严格)"() -> ("Selection Start"=w540:T1)  [unwired: 2 in, 2 out]
                    n398 = Unbundle By Name(w540) -> ("Row"=w539:i32)
                    n399 = property on="表格" class="Tbl (严格)"() -> ("Value"=w541:string[][])  [unwired: 2 in, 2 out]
                    n400 = Number To Decimal String(number=w539) -> (decimal integer string=w543:string)  [unwired: 1 in]
                    n401 = Index Array(array=w541, index (row)=w539, index (col)=0 ("禁用的索引 (列)")) -> (element=w537:string)
                    n402 = String Subset(string=w537, length (rest)=10 ("长度（剩余）")) -> (substring=w536:string)  [unwired: 1 in]
                    n403 = invoke on="控件配置文件" class="Tbl (严格)" method="Set Cell Value"("X Index"=1 ("X索引"), "Y Index"=w535, "Value"=w543) -> ()  [unwired: 3 in, 6 out]
                    n404 = property on="布尔 2" class="Bool (严格)"("Caption.Text"=w536) -> ()  [unwired: 2 in, 2 out]
                    n405 = property on="布控2设置" class="Str"("Val(Sgnl)"=w536) -> ()  [unwired: 2 in, 2 out]
                    n406 = invoke on="控件配置文件" class="Tbl (严格)" method="Set Cell Value"("X Index"=0 ("X索引"), "Y Index"=w535, "Value"=w536) -> ()  [unwired: 3 in, 6 out]
                  }
                  frame "关联到布控3" {
                    w546 = T9 4 items=["刷新间隔", "波特率", "布尔1设置项", "布尔2设置项", "布尔3设置项", "布尔4设置项", "布尔5设置项", "布尔6设置项", "布尔7设置项", "布尔8设置项", "显控1设置", "显控2设置", "显控3设置", "显控4设置", "显控5设置", "显控6设置", "显控7设置", "显控8设置", "显控9设置", "显控10设置", "显控11设置", "显控12设置", "设控1设置", "设控2设置", "设控3设置", "设控4设置", "设控5设置", "设控6设置", "设控7设置", "设控8设置", "曲线1设置", "曲线2设置", "曲线3设置", "曲线4设置", "曲线5设置", "曲线6设置", "曲线7设置", "曲线8设置", "曲线9设置", "曲线10设置", "曲线11设置", "曲线12设置", "曲线13设置", "曲线14设置", "曲线15设置", "曲线16设置", "曲线17设置", "曲线18设置", "曲线19设置", "曲线20设置", "曲线21设置", "曲线22设置", "曲线23设置", "曲线24设置", "曲线25设置", "曲线26设置", "曲线27设置", "曲线28设置", "曲线29设置", "曲线30设置", "曲线31设置", "曲线32设置", "曲线33设置", "曲线34设置", "曲线35设置", "曲线36设置", "曲线37设置", "曲线38设置", "曲线39设置", "曲线40设置", "曲线41设置", "曲线42设置", "曲线43设置", "曲线44设置", "曲线45设置", "曲线46设置", "曲线47设置", "曲线48设置", "曲线49设置", "曲线50设置", "曲线51设置", "曲线52设置", "曲线53设置", "曲线54设置", "曲线55设置", "曲线56设置", "曲线57设置", "曲线58设置", "曲线59设置", "曲线60设置", "曲线61设置", "曲线62设置", "曲线63设置", "曲线64设置", "ID值", "数据模式"] ("DataInitDef")
                    n407 = property on="表格" class="Tbl (严格)"() -> ("Selection Start"=w551:T1)  [unwired: 2 in, 2 out]
                    n408 = Unbundle By Name(w551) -> ("Row"=w550:i32)
                    n409 = property on="表格" class="Tbl (严格)"() -> ("Value"=w552:string[][])  [unwired: 2 in, 2 out]
                    n410 = Number To Decimal String(number=w550) -> (decimal integer string=w554:string)  [unwired: 1 in]
                    n411 = Index Array(array=w552, index (row)=w550, index (col)=0 ("禁用的索引 (列)")) -> (element=w548:string)
                    n412 = String Subset(string=w548, length (rest)=10 ("长度（剩余）")) -> (substring=w547:string)  [unwired: 1 in]
                    n413 = invoke on="控件配置文件" class="Tbl (严格)" method="Set Cell Value"("X Index"=1 ("X索引"), "Y Index"=w546, "Value"=w554) -> ()  [unwired: 3 in, 6 out]
                    n414 = property on="布控3设置" class="Str"("Val(Sgnl)"=w547) -> ()  [unwired: 2 in, 2 out]
                    n415 = property on="布尔 3" class="Bool (严格)"("Caption.Text"=w547) -> ()  [unwired: 2 in, 2 out]
                    n416 = invoke on="控件配置文件" class="Tbl (严格)" method="Set Cell Value"("X Index"=0 ("X索引"), "Y Index"=w546, "Value"=w547) -> ()  [unwired: 3 in, 6 out]
                  }
                  frame "关联到布控4" {
                    w557 = T9 5 items=["刷新间隔", "波特率", "布尔1设置项", "布尔2设置项", "布尔3设置项", "布尔4设置项", "布尔5设置项", "布尔6设置项", "布尔7设置项", "布尔8设置项", "显控1设置", "显控2设置", "显控3设置", "显控4设置", "显控5设置", "显控6设置", "显控7设置", "显控8设置", "显控9设置", "显控10设置", "显控11设置", "显控12设置", "设控1设置", "设控2设置", "设控3设置", "设控4设置", "设控5设置", "设控6设置", "设控7设置", "设控8设置", "曲线1设置", "曲线2设置", "曲线3设置", "曲线4设置", "曲线5设置", "曲线6设置", "曲线7设置", "曲线8设置", "曲线9设置", "曲线10设置", "曲线11设置", "曲线12设置", "曲线13设置", "曲线14设置", "曲线15设置", "曲线16设置", "曲线17设置", "曲线18设置", "曲线19设置", "曲线20设置", "曲线21设置", "曲线22设置", "曲线23设置", "曲线24设置", "曲线25设置", "曲线26设置", "曲线27设置", "曲线28设置", "曲线29设置", "曲线30设置", "曲线31设置", "曲线32设置", "曲线33设置", "曲线34设置", "曲线35设置", "曲线36设置", "曲线37设置", "曲线38设置", "曲线39设置", "曲线40设置", "曲线41设置", "曲线42设置", "曲线43设置", "曲线44设置", "曲线45设置", "曲线46设置", "曲线47设置", "曲线48设置", "曲线49设置", "曲线50设置", "曲线51设置", "曲线52设置", "曲线53设置", "曲线54设置", "曲线55设置", "曲线56设置", "曲线57设置", "曲线58设置", "曲线59设置", "曲线60设置", "曲线61设置", "曲线62设置", "曲线63设置", "曲线64设置", "ID值", "数据模式"] ("DataInitDef")
                    n417 = property on="表格" class="Tbl (严格)"() -> ("Selection Start"=w563:T1)  [unwired: 2 in, 2 out]
                    n418 = Unbundle By Name(w563) -> ("Row"=w561:i32)
                    n419 = property on="表格" class="Tbl (严格)"() -> ("Value"=w564:string[][])  [unwired: 2 in, 2 out]
                    n420 = Number To Decimal String(number=w561) -> (decimal integer string=w565:string)  [unwired: 1 in]
                    n421 = Index Array(array=w564, index (row)=w561, index (col)=0 ("禁用的索引 (列)")) -> (element=w560:string)
                    n422 = String Subset(string=w560, length (rest)=10 ("长度（剩余）")) -> (substring=w559:string)  [unwired: 1 in]
                    n423 = invoke on="控件配置文件" class="Tbl (严格)" method="Set Cell Value"("X Index"=1 ("X索引"), "Y Index"=w557, "Value"=w565) -> ()  [unwired: 3 in, 6 out]
                    n424 = property on="布尔 4" class="Bool (严格)"("Caption.Text"=w559) -> ()  [unwired: 2 in, 2 out]
                    n425 = property on="布控4设置" class="Str"("Val(Sgnl)"=w559) -> ()  [unwired: 2 in, 2 out]
                    n426 = invoke on="控件配置文件" class="Tbl (严格)" method="Set Cell Value"("X Index"=0 ("X索引"), "Y Index"=w557, "Value"=w559) -> ()  [unwired: 3 in, 6 out]
                  }
                  frame "关联到布控5" {
                    w568 = T9 6 items=["刷新间隔", "波特率", "布尔1设置项", "布尔2设置项", "布尔3设置项", "布尔4设置项", "布尔5设置项", "布尔6设置项", "布尔7设置项", "布尔8设置项", "显控1设置", "显控2设置", "显控3设置", "显控4设置", "显控5设置", "显控6设置", "显控7设置", "显控8设置", "显控9设置", "显控10设置", "显控11设置", "显控12设置", "设控1设置", "设控2设置", "设控3设置", "设控4设置", "设控5设置", "设控6设置", "设控7设置", "设控8设置", "曲线1设置", "曲线2设置", "曲线3设置", "曲线4设置", "曲线5设置", "曲线6设置", "曲线7设置", "曲线8设置", "曲线9设置", "曲线10设置", "曲线11设置", "曲线12设置", "曲线13设置", "曲线14设置", "曲线15设置", "曲线16设置", "曲线17设置", "曲线18设置", "曲线19设置", "曲线20设置", "曲线21设置", "曲线22设置", "曲线23设置", "曲线24设置", "曲线25设置", "曲线26设置", "曲线27设置", "曲线28设置", "曲线29设置", "曲线30设置", "曲线31设置", "曲线32设置", "曲线33设置", "曲线34设置", "曲线35设置", "曲线36设置", "曲线37设置", "曲线38设置", "曲线39设置", "曲线40设置", "曲线41设置", "曲线42设置", "曲线43设置", "曲线44设置", "曲线45设置", "曲线46设置", "曲线47设置", "曲线48设置", "曲线49设置", "曲线50设置", "曲线51设置", "曲线52设置", "曲线53设置", "曲线54设置", "曲线55设置", "曲线56设置", "曲线57设置", "曲线58设置", "曲线59设置", "曲线60设置", "曲线61设置", "曲线62设置", "曲线63设置", "曲线64设置", "ID值", "数据模式"] ("DataInitDef")
                    n427 = property on="表格" class="Tbl (严格)"() -> ("Selection Start"=w576:T1)  [unwired: 2 in, 2 out]
                    n428 = Unbundle By Name(w576) -> ("Row"=w575:i32)
                    n429 = property on="表格" class="Tbl (严格)"() -> ("Value"=w577:string[][])  [unwired: 2 in, 2 out]
                    n430 = Number To Decimal String(number=w575) -> (decimal integer string=w578:string)  [unwired: 1 in]
                    n431 = Index Array(array=w577, index (row)=w575, index (col)=0 ("禁用的索引 (列)")) -> (element=w574:string)
                    n432 = String Subset(string=w574, length (rest)=10 ("长度（剩余）")) -> (substring=w573:string)  [unwired: 1 in]
                    n433 = invoke on="控件配置文件" class="Tbl (严格)" method="Set Cell Value"("X Index"=1 ("X索引"), "Y Index"=w568, "Value"=w578) -> ()  [unwired: 3 in, 6 out]
                    n434 = property on="布尔 5" class="Bool (严格)"("Caption.Text"=w573) -> ()  [unwired: 2 in, 2 out]
                    n435 = property on="布控5设置" class="Str"("Val(Sgnl)"=w573) -> ()  [unwired: 2 in, 2 out]
                    n436 = invoke on="控件配置文件" class="Tbl (严格)" method="Set Cell Value"("X Index"=0 ("X索引"), "Y Index"=w568, "Value"=w573) -> ()  [unwired: 3 in, 6 out]
                  }
                  frame "关联到布控6" {
                    w579 = T9 7 items=["刷新间隔", "波特率", "布尔1设置项", "布尔2设置项", "布尔3设置项", "布尔4设置项", "布尔5设置项", "布尔6设置项", "布尔7设置项", "布尔8设置项", "显控1设置", "显控2设置", "显控3设置", "显控4设置", "显控5设置", "显控6设置", "显控7设置", "显控8设置", "显控9设置", "显控10设置", "显控11设置", "显控12设置", "设控1设置", "设控2设置", "设控3设置", "设控4设置", "设控5设置", "设控6设置", "设控7设置", "设控8设置", "曲线1设置", "曲线2设置", "曲线3设置", "曲线4设置", "曲线5设置", "曲线6设置", "曲线7设置", "曲线8设置", "曲线9设置", "曲线10设置", "曲线11设置", "曲线12设置", "曲线13设置", "曲线14设置", "曲线15设置", "曲线16设置", "曲线17设置", "曲线18设置", "曲线19设置", "曲线20设置", "曲线21设置", "曲线22设置", "曲线23设置", "曲线24设置", "曲线25设置", "曲线26设置", "曲线27设置", "曲线28设置", "曲线29设置", "曲线30设置", "曲线31设置", "曲线32设置", "曲线33设置", "曲线34设置", "曲线35设置", "曲线36设置", "曲线37设置", "曲线38设置", "曲线39设置", "曲线40设置", "曲线41设置", "曲线42设置", "曲线43设置", "曲线44设置", "曲线45设置", "曲线46设置", "曲线47设置", "曲线48设置", "曲线49设置", "曲线50设置", "曲线51设置", "曲线52设置", "曲线53设置", "曲线54设置", "曲线55设置", "曲线56设置", "曲线57设置", "曲线58设置", "曲线59设置", "曲线60设置", "曲线61设置", "曲线62设置", "曲线63设置", "曲线64设置", "ID值", "数据模式"] ("DataInitDef")
                    n437 = property on="表格" class="Tbl (严格)"() -> ("Selection Start"=w587:T1)  [unwired: 2 in, 2 out]
                    n438 = Unbundle By Name(w587) -> ("Row"=w586:i32)
                    n439 = property on="表格" class="Tbl (严格)"() -> ("Value"=w588:string[][])  [unwired: 2 in, 2 out]
                    n440 = Number To Decimal String(number=w586) -> (decimal integer string=w589:string)  [unwired: 1 in]
                    n441 = Index Array(array=w588, index (row)=w586, index (col)=0 ("禁用的索引 (列)")) -> (element=w585:string)
                    n442 = String Subset(string=w585, length (rest)=10 ("长度（剩余）")) -> (substring=w584:string)  [unwired: 1 in]
                    n443 = invoke on="控件配置文件" class="Tbl (严格)" method="Set Cell Value"("X Index"=1 ("X索引"), "Y Index"=w579, "Value"=w589) -> ()  [unwired: 3 in, 6 out]
                    n444 = property on="布尔 6" class="Bool (严格)"("Caption.Text"=w584) -> ()  [unwired: 2 in, 2 out]
                    n445 = property on="布控6设置" class="Str"("Val(Sgnl)"=w584) -> ()  [unwired: 2 in, 2 out]
                    n446 = invoke on="控件配置文件" class="Tbl (严格)" method="Set Cell Value"("X Index"=0 ("X索引"), "Y Index"=w579, "Value"=w584) -> ()  [unwired: 3 in, 6 out]
                  }
                  frame "关联到布控7" {
                    w590 = T9 8 items=["刷新间隔", "波特率", "布尔1设置项", "布尔2设置项", "布尔3设置项", "布尔4设置项", "布尔5设置项", "布尔6设置项", "布尔7设置项", "布尔8设置项", "显控1设置", "显控2设置", "显控3设置", "显控4设置", "显控5设置", "显控6设置", "显控7设置", "显控8设置", "显控9设置", "显控10设置", "显控11设置", "显控12设置", "设控1设置", "设控2设置", "设控3设置", "设控4设置", "设控5设置", "设控6设置", "设控7设置", "设控8设置", "曲线1设置", "曲线2设置", "曲线3设置", "曲线4设置", "曲线5设置", "曲线6设置", "曲线7设置", "曲线8设置", "曲线9设置", "曲线10设置", "曲线11设置", "曲线12设置", "曲线13设置", "曲线14设置", "曲线15设置", "曲线16设置", "曲线17设置", "曲线18设置", "曲线19设置", "曲线20设置", "曲线21设置", "曲线22设置", "曲线23设置", "曲线24设置", "曲线25设置", "曲线26设置", "曲线27设置", "曲线28设置", "曲线29设置", "曲线30设置", "曲线31设置", "曲线32设置", "曲线33设置", "曲线34设置", "曲线35设置", "曲线36设置", "曲线37设置", "曲线38设置", "曲线39设置", "曲线40设置", "曲线41设置", "曲线42设置", "曲线43设置", "曲线44设置", "曲线45设置", "曲线46设置", "曲线47设置", "曲线48设置", "曲线49设置", "曲线50设置", "曲线51设置", "曲线52设置", "曲线53设置", "曲线54设置", "曲线55设置", "曲线56设置", "曲线57设置", "曲线58设置", "曲线59设置", "曲线60设置", "曲线61设置", "曲线62设置", "曲线63设置", "曲线64设置", "ID值", "数据模式"] ("DataInitDef")
                    n447 = property on="表格" class="Tbl (严格)"() -> ("Selection Start"=w598:T1)  [unwired: 2 in, 2 out]
                    n448 = Unbundle By Name(w598) -> ("Row"=w597:i32)
                    n449 = property on="表格" class="Tbl (严格)"() -> ("Value"=w599:string[][])  [unwired: 2 in, 2 out]
                    n450 = Number To Decimal String(number=w597) -> (decimal integer string=w600:string)  [unwired: 1 in]
                    n451 = Index Array(array=w599, index (row)=w597, index (col)=0 ("禁用的索引 (列)")) -> (element=w596:string)
                    n452 = String Subset(string=w596, length (rest)=10 ("长度（剩余）")) -> (substring=w595:string)  [unwired: 1 in]
                    n453 = invoke on="控件配置文件" class="Tbl (严格)" method="Set Cell Value"("X Index"=1 ("X索引"), "Y Index"=w590, "Value"=w600) -> ()  [unwired: 3 in, 6 out]
                    n454 = property on="布尔 7" class="Bool (严格)"("Caption.Text"=w595) -> ()  [unwired: 2 in, 2 out]
                    n455 = property on="布控7设置" class="Str"("Val(Sgnl)"=w595) -> ()  [unwired: 2 in, 2 out]
                    n456 = invoke on="控件配置文件" class="Tbl (严格)" method="Set Cell Value"("X Index"=0 ("X索引"), "Y Index"=w590, "Value"=w595) -> ()  [unwired: 3 in, 6 out]
                  }
                  frame "关联到布控8" {
